vi "Stopping Event.vi"(11 "User Event in":refnum<user-event>) -> (3 "User Event out":refnum<user-event>)   [LabVIEW 2015, in "Command Handler.lvlib" / "Command Handler.lvclass"]
uses:
  Command Handler.lvclass
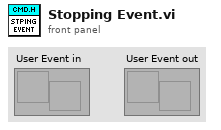
[diagram p1: front panel]
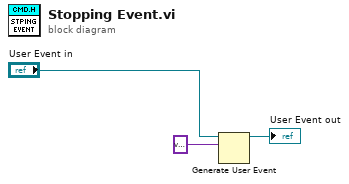
[diagram p0: block diagram]
diagram:
  n1 = Generate User Event(user event="User Event in", event data cluster=variant ("event data")) -> (user event out=→"User Event out":refnum<user-event>)  [unwired: 2 in, 1 out]
